vi "Start Or Stop.vi"(8 "error in (no error)":errorcluster, 10 "MM Gui Updates In":refnum<queue>, 11 "MM Button Events In":refnum<notifier>) -> (0 "error out":errorcluster, 1 "Start or Stop":T1, 2 "MM Gui Updates Out":refnum<queue>, 3 "Button Events Out":refnum<notifier>)   [LabVIEW 2009]
uses:
  Mixed Mode Button Events Message.ctl
  Mixed Mode Button Events.ctl
  Mixed Mode Widget Button States.ctl
  Mixed Mode Control Type.ctl
  Mixed Mode Gui Update Msg.ctl
  Mixed Mode GUI Update Type.ctl
  Target.ctl
  Data Access Objects/Metadata/LBCB Number.ctl
  Accepted or Declined.ctl
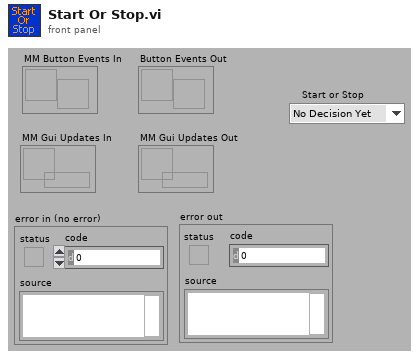
[diagram p1: front panel]
types:
  T1 = typedef "Accepted or Declined.ctl" = enum16{"No Decision Yet", "Accepted", "Declined"}
  T2 = typedef "Mixed Mode Gui Update Msg.ctl" = cluster{"MM GUI Update Type":T3, "Targets":T4[], "State":bool, "Step":string}
  T3 = typedef "Mixed Mode GUI Update Type.ctl" = enum16{"Nop", "Targets", "Accept.Blink", "Start.Blink", "TestStats", "Control.Enabled", "StartTestTimer", "RunInputFile"}
  T4 = typedef "Target.ctl" = cluster{"LBCB Number":T5, "DOF Vectors":enum16{" ", "Dx", "Dy", "Dz", "Rx", "Ry", "Rz", "Fx", "Fy", "Fz", "Mx", "My", "Mz"}, "Amount":dbl}
  T5 = typedef "LBCB Number.ctl" = enum16{"LBCB1", "LBCB2"}
  T6 = typedef "Mixed Mode Button Events Message.ctl" = cluster{"MM Control Events":T7, "Button States":T8}
  T7 = typedef "Mixed Mode Button Events.ctl" = enum16{"Propose.Accept", "Propose.Decline", "Execute.Start", "Execute.Stop", "TargetChange", "InputFile.Load", "InputFile.Reset", "InputFile.Pause", "InputFile.Run", "CartesianType.Changed", "NCTP.ConnectToServer", "Application.Stop", "Control.Enabled", "Control.Disabled", "ControlType.Changed", "Nop"}
  T8 = typedef "Mixed Mode Widget Button States.ctl" = cluster{"Auto-Start Enabled":bool, "Auto-Accept Enabled":bool, "Exit Requested":bool, "Mixed Mode Control Type":T9, "Input File Loaded":bool, "Input File Running":bool}
  T9 = typedef "Mixed Mode Control Type.ctl" = enum32{"Manual", "Input File", "NTCP"}
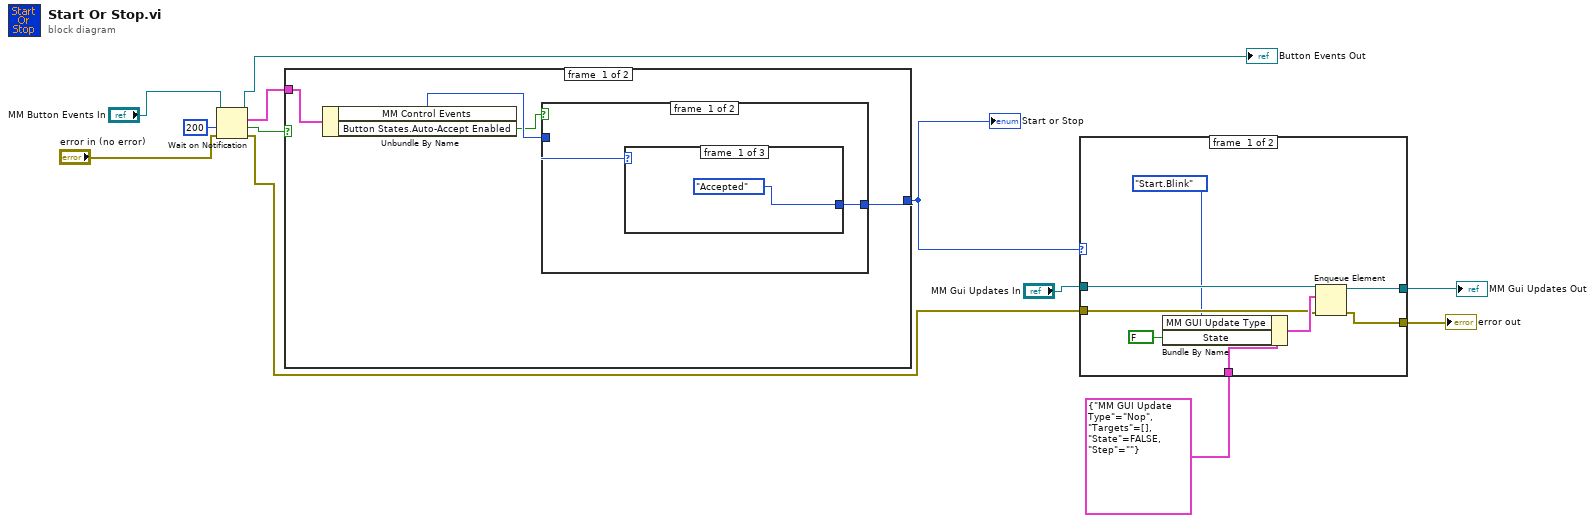
[diagram p0: block diagram]
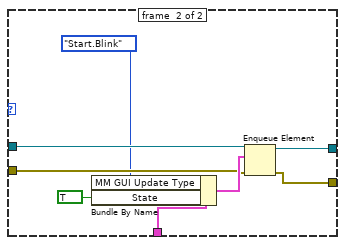
[diagram p2: hidden frame]
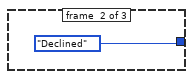
[diagram p3: hidden frame]
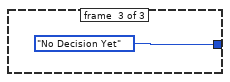
[diagram p4: hidden frame]
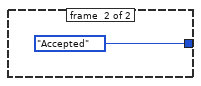
[diagram p5: hidden frame]
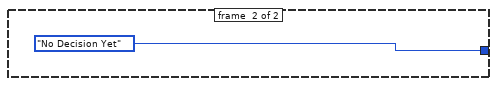
[diagram p6: hidden frame]
diagram:
  n1 = Wait on Notification(notifier="MM Button Events In", timeout in ms (-1)=200, error in (no error)="error in (no error)") -> (notifier out=→"Button Events Out":refnum<notifier>, notification=w7:T6, timed out?=w8:bool, error out=w2:errorcluster)  [unwired: 1 in]
  n2 = case shown="False" w8 {
    tunnel: w7 -> [w16 _]
    tunnel: [w13 Accepted_or_Declined."No Decision Yet" ("Accepted or Declined")] -> w1
    frame #0 {
      n3 = Unbundle By Name(w16) -> ("MM Control Events"=w15:T7, "Button States.Auto-Accept Enabled"=w14:bool)
      n4 = case shown="False" w14 {
        tunnel: w15 -> [w18 _]
        tunnel: [w17 Accepted_or_Declined."Accepted" ("Accepted or Declined")] -> w13
        frame #0 {
          n5 = case shown="\"TargetChange\", Default" w18 {
            tunnel: [Accepted_or_Declined."Accepted" ("Accepted or Declined") Accepted_or_Declined."Declined" ("Accepted or Declined") Accepted_or_Declined."No Decision Yet" ("Accepted or Declined")] -> w17
            frame #0 {
            }
            frame #1 {
            }
            frame #2 {
            }
          }
        }
        frame #1 {
        }
      }
    }
    frame #1 {
    }
  }
  "Start or Stop" <- w1
  n6 = case shown="\"No Decision Yet\"" w1 {
    tunnel: "MM Gui Updates In" -> [w31 w39]
    tunnel: T2 {"MM GUI Update Type"=enum."Nop", "Targets"=[], "State"=FALSE, "Step"=""} ("element") -> [w30 w38]
    tunnel: [w28 w36] -> w4
    tunnel: [w27 w35] -> w3
    tunnel: w2 -> [w26 w34]
    frame #0 {
      n7 = Bundle By Name(cluster=w30, "MM GUI Update Type"=Mixed_Mode_GUI_Update_Type."Start.Blink", "State"=FALSE) -> (w29:T2)
      n8 = Enqueue Element(queue=w31, element=w29, error in (no error)=w26) -> (queue out=w28:refnum<queue>, error out=w27:errorcluster)  [unwired: 1 in, 1 out]
    }
    frame #1 {
      n9 = Bundle By Name(cluster=w38, "MM GUI Update Type"=Mixed_Mode_GUI_Update_Type."Start.Blink", "State"=TRUE) -> (w37:T2)
      n10 = Enqueue Element(queue=w39, element=w37, error in (no error)=w34) -> (queue out=w36:refnum<queue>, error out=w35:errorcluster)  [unwired: 1 in, 1 out]
    }
  }
  "MM Gui Updates Out" <- w4
  "error out" <- w3
